vi "NumDecoder.vi"(1 "Byte Array":u8[](array[numeric]), 2 "Method":T1(ring)) -> (0 "Number":dbl format="%#_13g")   [LabVIEW 2014]
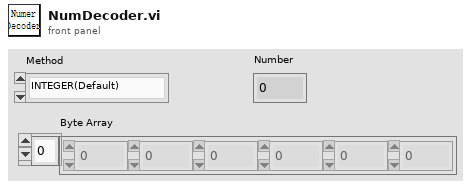
[diagram p1: front panel]
types:
  T1 = enum16{"INTEGER(Default)", "SIGNED_5", "UNSIGNED_7", "SIGNED_10", "SIGNED_12"}
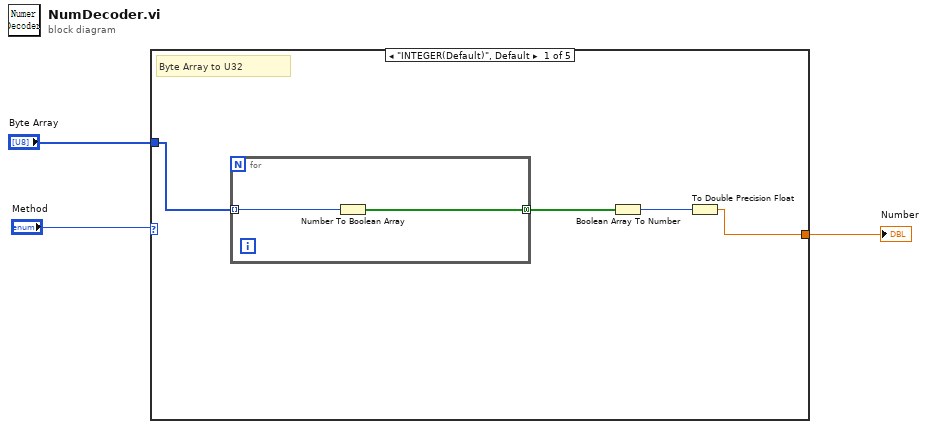
[diagram p0: block diagram]
diagram:
  n1 = case shown="\"INTEGER(Default)\", Default" "Method" {
    tunnel: "Byte Array" -> [w7 _ _ _ _]
    tunnel: [w4 _ _ _ _] -> w1
    frame "INTEGER(Default)", Default {
      # "Byte Array to U32"
      n2 = for {
        tunnel: w7 -> [w9] mode=indexing
        tunnel: [w8] -> w6 mode=concatenating
        n3 = Number To Boolean Array(number=w9) -> (Boolean array=w8:bool[])
      }
      n4 = Boolean Array To Number(Boolean array=w6) -> (number=w5:u32)
      n5 = To Double Precision Float(number=w5) -> (double precision float=w4:dbl)
    }
    frame "SIGNED_5" {
      # "(-16, 16)"
    }
    frame "UNSIGNED_7" {
      # "(0, 90)"
    }
    frame "SIGNED_10" {
      # "(-360, 360)"
    }
    frame "SIGNED_12" {
      # "(-2000, 2000)"
    }
  }
  "Number" <- w1
